vi "AfterPage2_GenCD.vi"(10 "MetaDataObj":refnum<class "MetaDataObj.lvclass">, 11 "User Project":refnum<vi>) -> ()   [LabVIEW 2015, in "NIVS_CDW_MetaDataObj.lvclass"]
uses:
  NIVS_CDW_MetaDataObj.lvclass
  <resource>/dialog/NewProjectWizard/MetaDataObj/MetaDataObj.lvclass
  NIVS_CDW_MetaDataObj.lvclass/NIVS_CDW_MetaDataObj.ctl
  <resource>/dialog/NewProjectWizard/MetaDataObj/MetaDataObj.lvclass/MetaDataObj.ctl
  <resource>/dialog/NewProjectWizard/MetaDataObj/Accessors/Read Project Root.vi
  <resource>/dialog/NewProjectWizard/MetaDataObj/Accessors/Read Project Name.vi
panel:
  # "Make a copy of this template to implement your own AfterPage2NoUI scripting VI for your custom template/sample project."
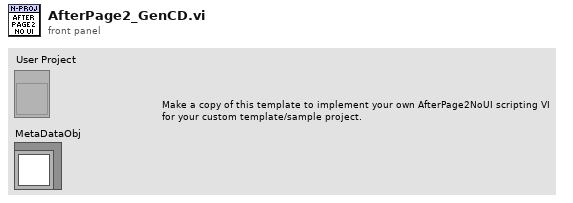
[diagram p1: front panel]
types:
  T1 = typedef "CD Wizard - Internal data.ctl" = cluster{"Common Information":cluster{"CD Name":string, "CD Target Folder":path, "CD Execution Mode":T2, "CD GUID":string, "Max Occurrences":u32}, "Extra Pages":T3[], "References":cluster{"System Explorer Library":refnum<vi>, "Shared Library":refnum<vi>, "Engine Library":refnum<vi>}, "Menu Settings":cluster{"Insert CD in submenu":bool, "Parent Menu Name":string}}
  T2 = typedef "CD Wizard - Execution Mode.ctl" = enum16{"Asynchronous", "Inline HW Interface", "Inline Model Interface", "Inline Timing and Sync", "Asynchronous Timing and Sync"}
  T3 = typedef "CD Wizard - Extra Page Name and GUID.ctl" = cluster{"Page Name":string, "Page GUID":string}
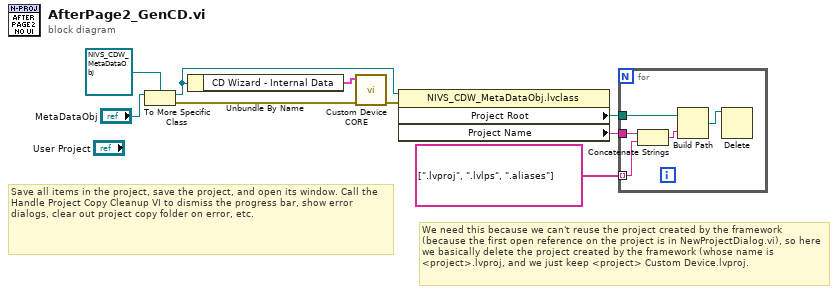
[diagram p0: block diagram]
diagram:
  # "We need this because we can't reuse the project created by the framework (because the first open reference on the project is in NewProjectDialog.vi), so here we basically delete the project created by the framework (whose name is <project>.lvproj, and we just keep <project> Custom Device.lvproj."
  # "Save all items in the project, save the project, and open its window. Call the Handle Project Copy Cleanup VI to dismiss the progress bar, show error dialogs, clear out project copy folder on error, etc."
  n1 = To More Specific Class(target class=refnum<class "NIVS_CDW_MetaDataObj.lvclass"> refnum ("NIVS_CDW_MetaDataObj.lvclass"), reference="MetaDataObj") -> (specific class reference=w7:refnum<class "NIVS_CDW_MetaDataObj.lvclass">, error out=w4:errorcluster)  [unwired: 1 in]
  n2 = Unbundle By Name(w7) -> ("CD Wizard - Internal Data"=w6:T1)
  n3 = call "Custom Device CORE.vi"("error in (no error)"=w4, "CD Wizard - Internal Data"=w6) -> ("error out"=w5:errorcluster)  [unwired: 9 in]
  n4 = property class="NIVS_CDW_MetaDataObj.lvclass"(reference=w7, error in=w5) -> ("Project Root"=w3:path, "Project Name"=w2:string)  [unwired: 2 out]
  n5 = for {
    tunnel: w3 -> [w14]
    tunnel: w2 -> [w13]
    tunnel: string[] [".lvproj", ".lvlps", ".aliases"] -> [w12] mode=indexing
    n6 = Concatenate Strings(w13, w12) -> (w11:string)
    n7 = Build Path(base path=w14, name or relative path=w11) -> (appended path=w10:path)
    n8 = Delete(path (use dialog)=w10) -> ()  [unwired: 4 in, 3 out]
  }
